vi "N-664 Send Command.vi"(0 "VISA Ref":refnum<visa-resource-name>, 2 "Wait for Reply?":bool, 7 "Error In":errorcluster, 11 "Command":string) -> (4 "VISA Ref Out":refnum<visa-resource-name>, 8 "Error Out":errorcluster, 15 "Response":string)   [LabVIEW 2016]
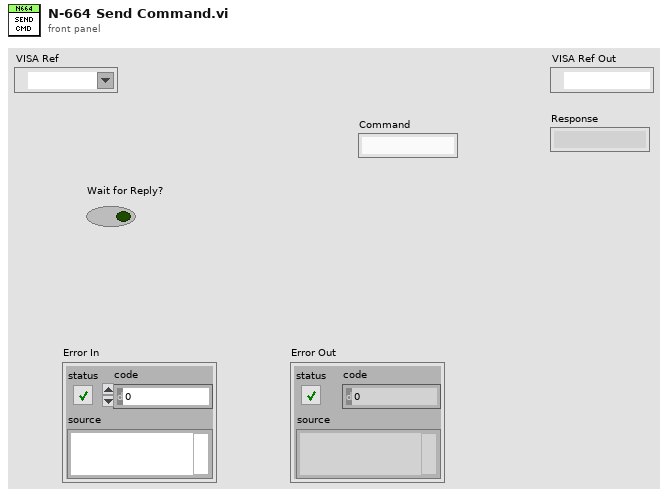
[diagram p1: front panel]
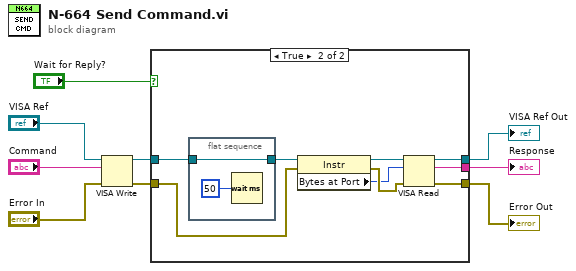
[diagram p0: block diagram]
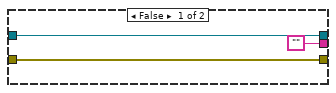
[diagram p2: hidden frame]
diagram:
  n1 = VISA Write(VISA resource name="VISA Ref", write buffer="Command", error in (no error)="Error In") -> (VISA resource name out=w9:refnum<visa-resource-name>, error out=w8:errorcluster)  [unwired: 1 out]
  n2 = case shown="True" "Wait for Reply?" {
    tunnel: w9 -> [w12 w17]
    tunnel: w8 -> [w11 w16]
    tunnel: [w12 w15] -> w6
    tunnel: [w11 w14] -> w5
    tunnel: ["" w13] -> w3
    frame False {
    }
    frame True {
      n3 = flat-sequence {
        tunnel: [w22] -> w20
        tunnel: w17 -> [w22]
        frame #0 {
          n4 = Wait (ms)(milliseconds to wait=u32 50) -> ()  [unwired: 1 out]
        }
      }
      n5 = property class="Instr"(reference=w20, error in=w16) -> (reference out=w18:refnum<visa-resource-name>, error out=w21:errorcluster, "Bytes at Port"=w19:u32)
      n6 = VISA Read(VISA resource name=w18, byte count=w19, error in (no error)=w21) -> (VISA resource name out=w15:refnum<visa-resource-name>, read buffer=w13:string, error out=w14:errorcluster)  [unwired: 1 out]
    }
  }
  "Response" <- w3
  "VISA Ref Out" <- w6
  "Error Out" <- w5
